vi "CRYSerial Control Lines Read visa Preinit.vi"(11 "COM port (1 = COM1, etc.)":i32=1 min=1 max=99) -> (3 "Line states (CTS, DSR, RI, DCD)":bool[](array[boolean]))   [LabVIEW 2013]
uses:
  Program/CRYRef nums global.vi
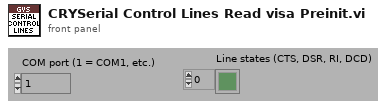
[diagram p1: front panel]
types:
  T1 = cluster{"COM port (1 = COM1, etc.)":i32, "VISA session (for class)":refnum<visa-resource-name>}[]
  T2 = cluster{"COM port (1 = COM1, etc.)":i32, "VISA session (for class)":refnum<visa-resource-name>}
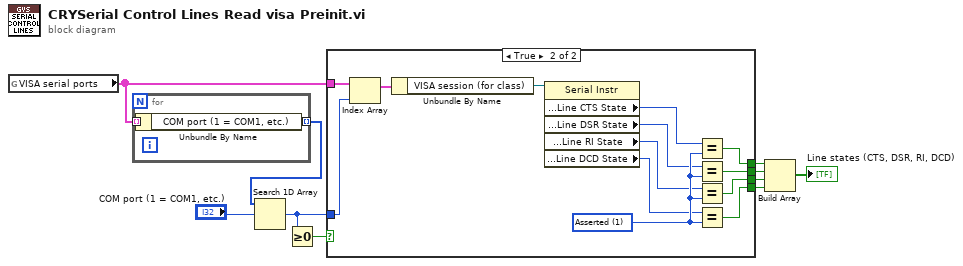
[diagram p0: block diagram]
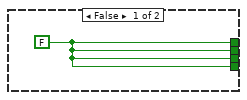
[diagram p2: hidden frame]
diagram:
  n1 = global read "CRYRef nums global.vi" "VISA serial ports"() -> (w1:T1)
  n2 = for {
    tunnel: w1 -> [w12] mode=indexing
    tunnel: [w11] -> w5 mode=indexing
    n3 = Unbundle By Name(w12) -> ("COM port (1 = COM1, etc.)"=w11:i32)
  }
  n4 = Search 1D Array(1D array=w5, element="COM port (1 = COM1, etc.)") -> (index of element=w2:i32)  [unwired: 1 out]
  n5 = Greater Or Equal To 0?(x=w2) -> (x >= 0?=w3:bool)
  n6 = case shown="True" w3 {
    tunnel: [w13 w21] -> w10
    tunnel: [w13 w20] -> w9
    tunnel: [w13 w19] -> w8
    tunnel: [w13 w18] -> w7
    tunnel: w2 -> [_ w16]
    tunnel: w1 -> [_ w17]
    frame False {
      w13 = FALSE
    }
    frame True {
      w26 = i16 1 items=["Unknown"=-1, "Unasserted"=0, "Asserted"=1] ("Modem Line Settings:Line DCD State")
      n7 = Index Array(array=w17, index=w16) -> (element=w15:T2)
      n8 = Unbundle By Name(w15) -> ("VISA session (for class)"=w14:refnum<visa-resource-name>)
      n9 = property class="Serial Instr"(reference=w14) -> ("Serial Settings:Modem Line Settings:Line CTS State"=w25:i16, "Serial Settings:Modem Line Settings:Line DSR State"=w24:i16, "Serial Settings:Modem Line Settings:Line RI State"=w23:i16, "Serial Settings:Modem Line Settings:Line DCD State"=w22:i16)  [unwired: 1 in, 2 out]
      n10 = Equal?(x=w25, y=w26) -> (x = y?=w21:bool)
      n11 = Equal?(x=w24, y=w26) -> (x = y?=w20:bool)
      n12 = Equal?(x=w23, y=w26) -> (x = y?=w19:bool)
      n13 = Equal?(x=w22, y=w26) -> (x = y?=w18:bool)
    }
  }
  n14 = Build Array(w10, w9, w8, w7) -> (→"Line states (CTS, DSR, RI, DCD)":bool[])
